vi "perpheralsInitialise.vi"(6 "No Legend":bool, 8 "Edge Axis Labels only":bool, 9 "Cols":u8, 10 "Rows":u8, 11 "GraphPeripheralsIn":T1[][](array[typedef])) -> (3 "GraphPeripheralsOut":T1[][](array[typedef]))   [LabVIEW 2012]
uses:
  graphPeripherals.ctl
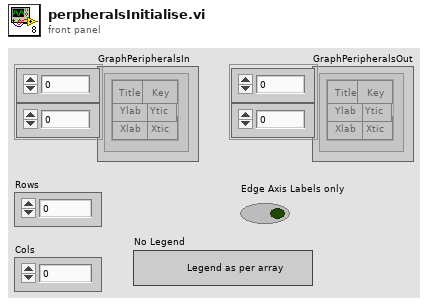
[diagram p1: front panel]
types:
  T1 = typedef "graphPeripherals.ctl" = cluster{"title":bool, "key":bool, "Xtic":bool, "Ytic":bool, "Xlab":bool, "Ylab":bool}
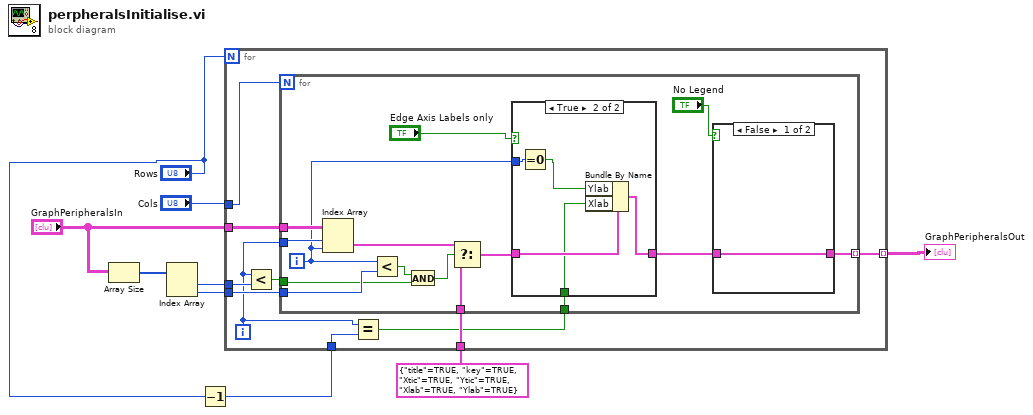
[diagram p0: block diagram]
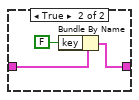
[diagram p2: hidden frame]
diagram:
  n1 = Array Size(array="GraphPeripheralsIn") -> (size(s)=w6:i32[])
  n2 = Index Array(array=w6) -> (element #1=w7:i32, element #2=w8:i32)  [unwired: 2 in]
  n3 = Decrement(x="Rows") -> (x-1=w1:u8)
  n4 = for {
    N: "Rows" -> [_]
    tunnel: "Cols" -> [w19]
    tunnel: "GraphPeripheralsIn" -> [w18]
    tunnel: [w17] -> w3 mode=indexing
    tunnel: w7 -> [w16]
    tunnel: w8 -> [w15]
    tunnel: T1 {"title"=TRUE, "key"=TRUE, "Xtic"=TRUE, "Ytic"=TRUE, "Xlab"=TRUE, "Ylab"=TRUE} ("Peripherals") -> [w13]
    tunnel: w1 -> [w12]
    i -> [w11]
    n5 = Less?(x=w11, y=w16) -> (x < y?=w14:bool)
    n6 = Equal?(x=w11, y=w12) -> (x = y?=w10:bool)
    n7 = for {
      N: w19 -> [_]
      tunnel: w18 -> [w34]
      tunnel: w11 -> [w33]
      tunnel: [w20] -> w17 mode=indexing
      tunnel: w15 -> [w32]
      tunnel: w14 -> [w30]
      tunnel: w13 -> [w27]
      tunnel: w10 -> [w23]
      i -> [w24]
      n8 = Index Array(array=w34, index (row)=w33, index (col)=w24) -> (element=w28:T1)
      n9 = Less?(x=w24, y=w32) -> (x < y?=w31:bool)
      n10 = And(x=w31, y=w30) -> (x .and. y?=w29:bool)
      n11 = Select(t=w28, s=w29, f=w27) -> (s? t:f=w25:T1)
      n12 = case shown="True" "Edge Axis Labels only" {
        tunnel: [w39 w40] -> w21
        tunnel: w25 -> [w39 w43]
        tunnel: w24 -> [_ w44]
        tunnel: w23 -> [_ w41]
        frame False {
        }
        frame True {
          n13 = Equal To 0?(x=w44) -> (x = 0?=w42:bool)
          n14 = Bundle By Name(cluster=w43, "Ylab"=w42, "Xlab"=w41) -> (w40:T1)
        }
      }
      n15 = case shown="False" "No Legend" {
        tunnel: w21 -> [w35 w38]
        tunnel: [w35 w37] -> w20
        frame False {
        }
        frame True {
          n16 = Bundle By Name(cluster=w38, "key"=FALSE) -> (w37:T1)
        }
      }
    }
  }
  "GraphPeripheralsOut" <- w3
